vi "FTW-Crypto-String-Verify.vi"(0 "Signed String":string, 5 "Regex to Match Signature":string="\"Signature\"(?:\\s*)?:(?:\\s*)?\"\\K(.*?)(?=\")", 7 "Public Verification Key":string, 11 "error in":errorcluster) -> (4 "Signature Verified":bool, 6 "Valid Verification Key Structure":bool, 8 "Found Signature":bool, 15 "error out":errorcluster)   [LabVIEW 2015]
panel:
  # "Inputs"
  # "Outputs"
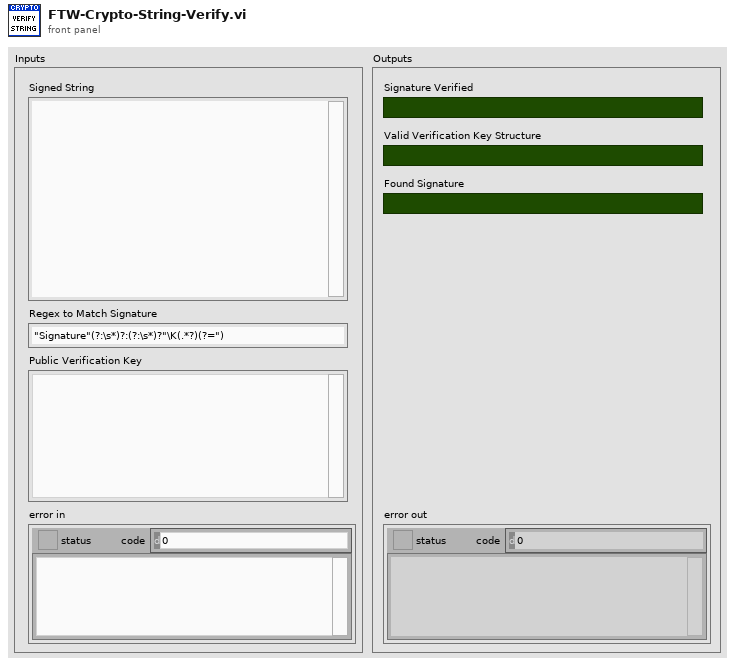
[diagram p1: front panel]
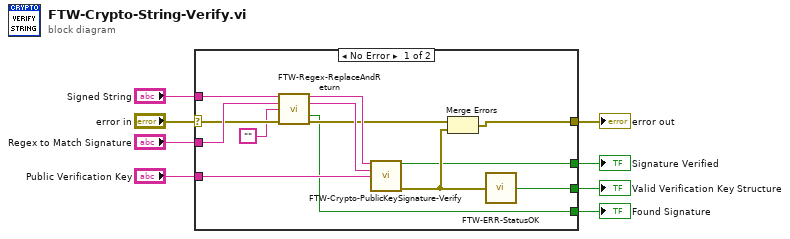
[diagram p0: block diagram]
diagram:
  n1 = case shown="No Error" "error in" {
    selector: "error in" -> [w15 w22]
    tunnel: [w12 w22] -> w8
    tunnel: "Signed String" -> [w18 _]
    tunnel: "Public Verification Key" -> [w20 _]
    tunnel: "Regex to Match Signature" -> [w19 _]
    tunnel: [w21 _] -> w3
    tunnel: [w9 _] -> w2
    tunnel: [w11 _] -> w1
    frame No Error {
      n2 = call "FTW-Regex-ReplaceAndReturn.vi"("String"=w18, "Search for (Regular Expression)"=w19, "Replace with"="", "error in"=w15) -> ("String out"=w17:string, "Original Match (replaced)"=w16:string, "Match Found?"=w9:bool, "error out"=w13:errorcluster)  [unwired: 7 in, 1 out]
      n3 = call "FTW-Crypto-PublicKeySignature-Verify.vi"("Data"=w17, "Hex Encoded Signature"=w16, "Public Key"=w20) -> ("Signature Verified"=w11:bool, "error out"=w14:errorcluster)  [unwired: 11 in]
      n4 = Merge Errors(w13, w14) -> (w12:errorcluster)
      n5 = call "FTW-ERR-StatusOK.vi"("error to check"=w14) -> ("Status OK?"=w21:bool)
    }
    frame Error {
    }
  }
  "error out" <- w8
  "Valid Verification Key Structure" <- w3
  "Found Signature" <- w2
  "Signature Verified" <- w1
